vi "Flock_FormatErrorMsg.vi"(8 "error in (no error)":errorcluster, 11 "initial string":string) -> (2 "String":string, 3 "code":i32)   [LabVIEW 2014, in "Flock_ErrorHandling.lvlib"]
uses:
  Flock_ErrorHandling.lvlib
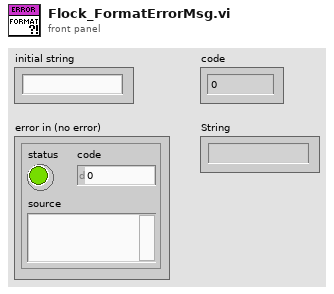
[diagram p1: front panel]
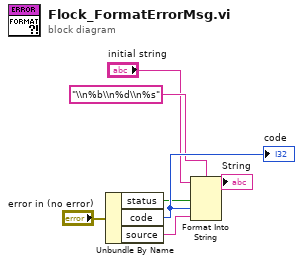
[diagram p0: block diagram]
diagram:
  n1 = Unbundle By Name("error in (no error)") -> ("status"=w3:bool, "code"=w7:i32, "source"=w6:string)
  "code" <- w7
  n2 = Format Into String(format string="\\n%b\\n%d\\n%s", initial string="initial string", w3, w7, w6) -> (resulting string=→"String":string)  [unwired: 1 in, 1 out]
